vi "Test.vi"() -> ()   [LabVIEW 2022 SP3, in "FHPP.lvclass"]
uses:
  FHPP.lvclass
  Operating Mode.ctl
  DIR.ctl
  CCON.ctl
  Setpoints.ctl
  FHPP.lvclass/FHPP.ctl
panel:
  in  "data value 3":T1 {"Setpoint" max=100; "Vel/VelRamp (%)" max=100}
  in  "data value 2":T2
  in  "data value":T4
  in  "stop":bool
  in  "Operating Mode 2":T3
  out "Operating Mode":T3
  out "error out 2":errorcluster
  out "error out":errorcluster
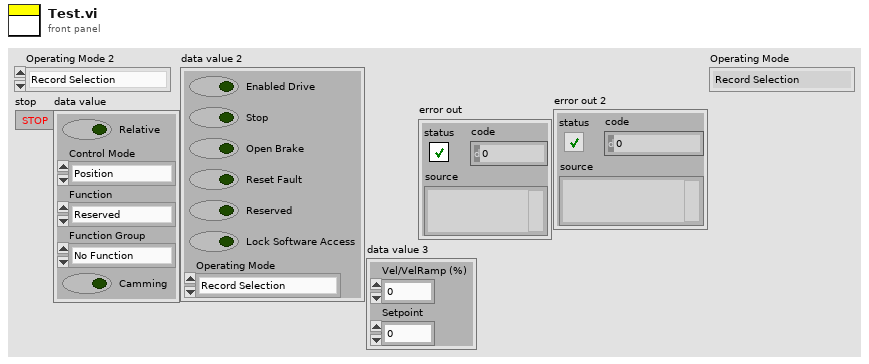
[diagram p1: front panel]
types:
  T1 = typedef "FHPP.lvclass/Setpoints.ctl" = cluster{"Vel/VelRamp (%)":u8, "Setpoint":u32}
  T2 = typedef "FHPP.lvclass/CCON.ctl" = cluster{"Enabled Drive":bool, "Stop":bool, "Open Brake":bool, "Reset Fault":bool, "Reserved":bool, "Lock Software Access":bool, "Operating Mode":T3}
  T3 = typedef "FHPP.lvclass/Operating Mode.ctl" = enum16{"Record Selection", "Direct Mode", "Reserved 1", "Reserved 2"}
  T4 = typedef "FHPP.lvclass/DIR.ctl" = cluster{"Relative":bool, "Control Mode":enum8{"Position", "Force", "Velocity", "Reserved"}, "Function":enum8{"Reserved", "External Input", "External Input with  Cam", "Virtual Master with Cam"}, "Function Group":enum8{"No Function", "Reserver 1", "Reserved 2", "Reserved 3"}, "Camming":bool}
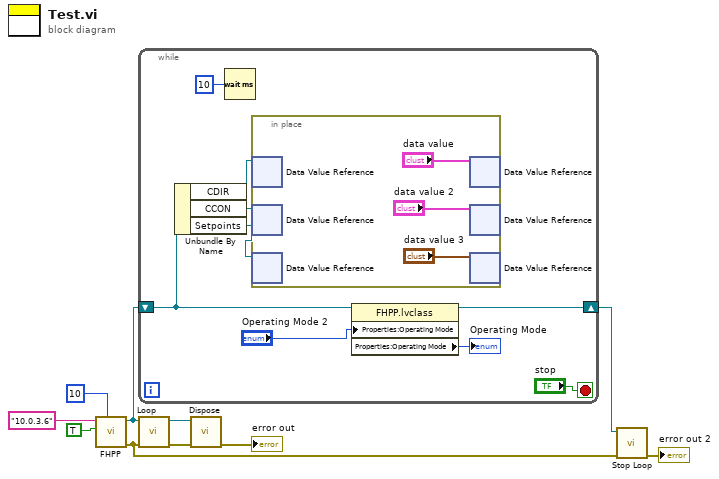
[diagram p0: block diagram]
diagram:
  n1 = call "FHPP.vi"("Cyle (ms)"=10, "Use FCT"=TRUE, "IP Address"="10.0.3.6") -> ("error out"=w5:errorcluster, "FHPP out"=w2:refnum<class "FHPP.lvclass">)  [unwired: 7 in]
  n2 = while {
    shift-right: [w19] -> w1
    shift-left: w2 -> [w14]
    stop <- "stop" stop-if-true
    n3 = Unbundle By Name(w14) -> ("CDIR"=w13:refnum<data-value>, "CCON"=w12:refnum<data-value>, "Setpoints"=w11:refnum<data-value>)
    n4 = Wait (ms)(milliseconds to wait=u32 10) -> ()  [unwired: 1 out]
    n5 = in-place {
      n6 = in-place-dvr #1(w13) -> ()  [unwired: 2 out]
      n7 = in-place-dvr #2(w12) -> ()  [unwired: 2 out]
      n8 = in-place-dvr #3(w11) -> ()  [unwired: 2 out]
      n9 = in-place-dvr #1("data value") -> ()  [unwired: 2 out]
      n10 = in-place-dvr #2("data value 2") -> ()  [unwired: 2 out]
      n11 = in-place-dvr #3("data value 3") -> ()  [unwired: 2 out]
    }
    n12 = property class="FHPP.lvclass"(reference=w14, "Properties:Operating Mode"="Operating Mode 2") -> (reference out=w19:refnum<class "FHPP.lvclass">, "Properties:Operating Mode"=→"Operating Mode":T3)  [unwired: 1 in, 1 out]
  }
  n13 = call-dynamic "Loop.vi"("error in (no error)"=w5, "FHPP in"=w2) -> ("error out"=w8:errorcluster, "FHPP out"=w7:refnum<class "FHPP.lvclass">)  [unwired: 8 in]
  n14 = call-dynamic "Dispose.vi"("error in (no error)"=w8, "FHPP in"=w7) -> ("error out"=→"error out":errorcluster)  [unwired: 9 in]
  n15 = call-dynamic "Stop Loop.vi"("error in (no error)"=w5, "FHPP in"=w1) -> ("error out"=→"error out 2":errorcluster)  [unwired: 9 in]
